vi "dataQ Terminal.vi"() -> ()   [LabVIEW 2024]
doc: "This example performs writes and reads on a serial port, as directed by the user. You can press the Write and Read buttons, and change the Read Count, while the example is running.\n\nThe parameters set for the serial port must match the parameters of the connected instrument or device. In this example, the Read Count parameter specifies the number of bytes that the serial port reads. If there were more bytes at the port than the specified number, those bytes would not be read. If there were less bytes at the port than the specified number, you would receive a timeout error.\n\nThis example expands upon the flow control options for XON and XOFF, allowing the user to choose those control characters. Also, the user can enable or disable a termination character. Some devices require a termination character in order to identify the end of command strings. Some devices send a termination character to signify the end of data to be read. This example shows how you can end the Read operation once a termination character is detected in the buffer and/or append a termination character at the end of the Write data."
uses:
  <vilib>/Instr/_visa.llb/VISA Configure Serial Port (Instr).vi
panel:
  out "Numeric":i32
  out "read buffer":string
  in  "Command List":string="stop\nencode 0\nslist 0 0\nslist 1 1\nsrate 6000\nps 2\ndec 1\ndeca 3\nnop\n"
  in  "2108 CDC Virtual COM":refnum<visa-resource-name>="COM3"
  # "Analog In\n\nencode 0\nslist 0 0\nslist 1 1\nsrate 6000\nps 2\ndec 1\ndeca 3\nnop"
  # "encode 0\nslist 0 0\nslist 1 1\nsrate 6000\nps 2\ndec 1\ndeca 3\nnop"
  # "encode 0 Enables the binary output mode (DEFAULT"
  # "info 0    Returns \"info 0 DATAQ\"\ninfo 1    Returns device model number (e.g.\"info 1 2008\")\ninfo 2    Returns firmware revision, 2 hex bytes (e.g. 6516 = 10110 for firmware revision 1.01)\ninfo 3    to info 4 Proprietary internal use for initial system verification\ninfo 5    <arg0>\n            Sets device description string arg0 (31 characters followed by null). Issued without <arg0> returns the \n            previously defined device description string. arg0 may be contained within quotation marks to included spaces \n            in device description. Model DI-2008 does not support info 5.\ninfo 6    Returns the instrument's serial number (left-most 8 digits only)\ninfo 7    to info 8 Proprietary internal use for initial system verification\ninfo 9    Returns the sample rate dividend value based upon current settings (see the srate command for details"
  # "0x60 = 96   FILL\n0x40 = 64  OFF\n0x20 = 32  DRAIN\n0x00 = 00  OFF"
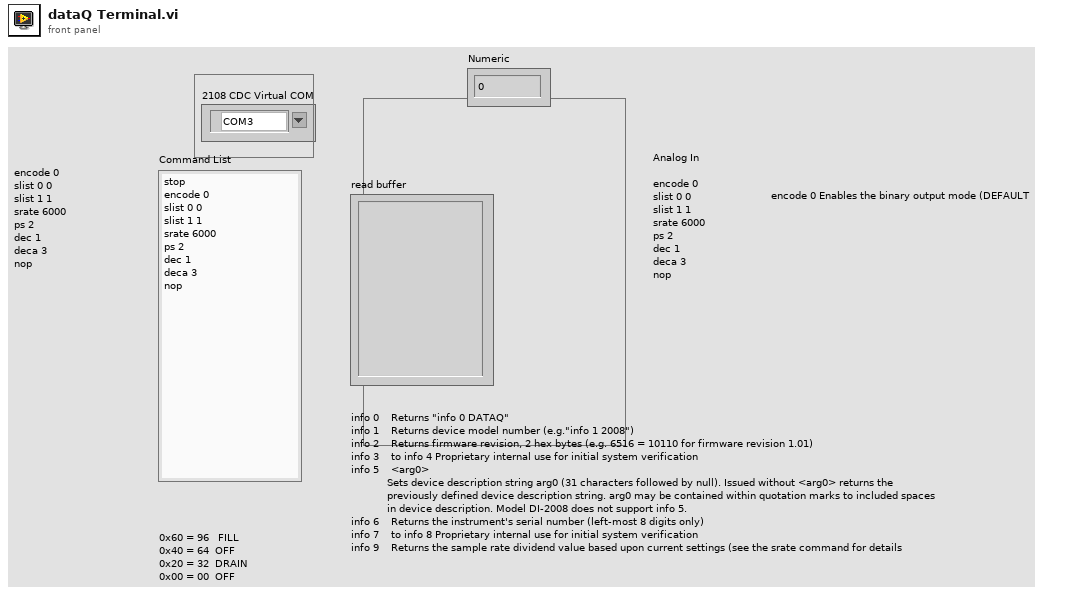
[diagram p1: front panel]
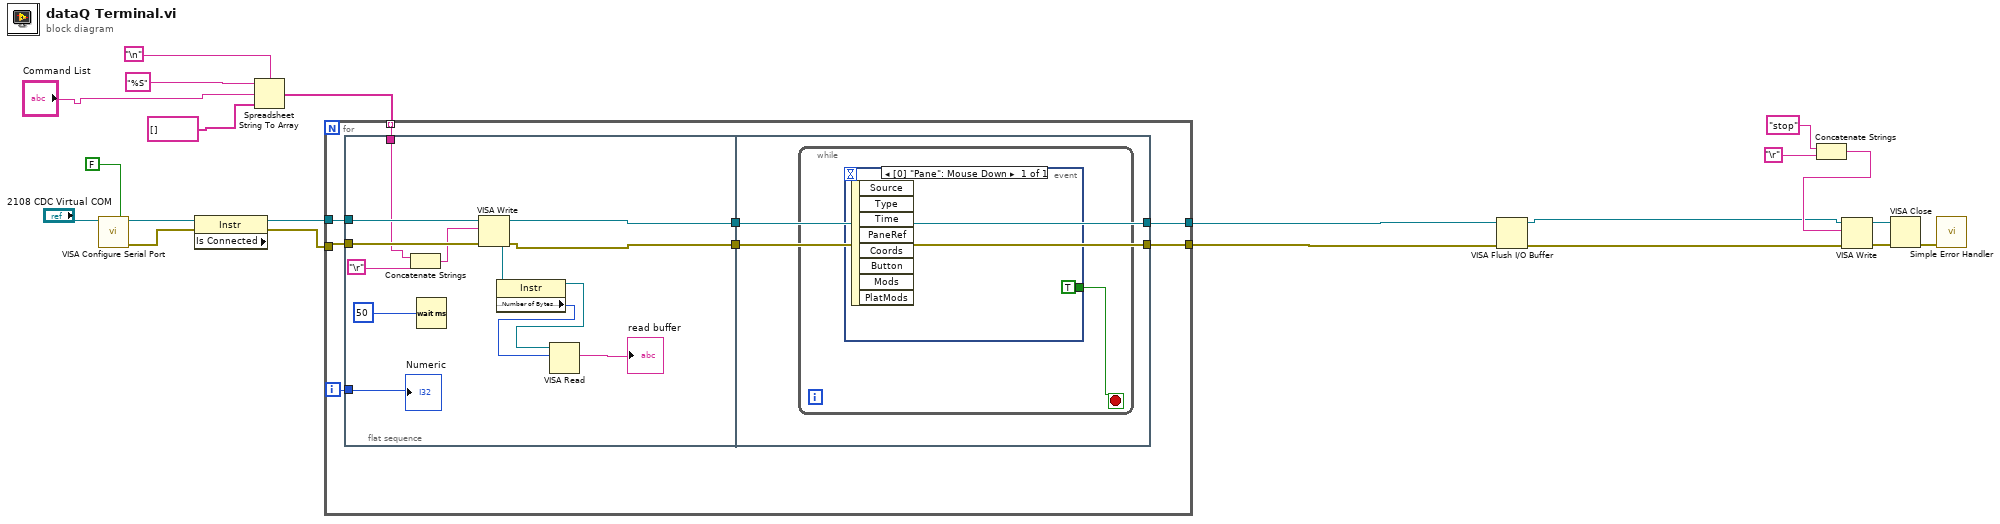
[diagram p0: block diagram]
diagram:
  n1 = call-poly "VISA Configure Serial Port"("VISA resource name"="2108 CDC Virtual COM", "Enable Termination\nChar (T)"=FALSE) -> ("VISA resource name out"=w19:refnum<visa-resource-name>, "error out"=w21:errorcluster)  [unwired: 8 in, 4 out]
  n2 = property class="Instr" props=["Is Connected"](reference=w19, error in=w21) -> (reference out=w5:refnum<visa-resource-name>, error out=w4:errorcluster)  [unwired: 1 out]
  n3 = Spreadsheet String To Array(delimiter (Tab)="\n", format string="%S", spreadsheet string="Command List", array type (2D Dbl)=string[] []) -> (array=w15:string[])
  n4 = for {
    tunnel: w15 -> [w27] mode=indexing
    tunnel: w5 -> [w29]
    tunnel: w4 -> [w28]
    tunnel: [w25] -> w7
    tunnel: [w26] -> w6
    i -> [w22]
    n5 = flat-sequence {
      tunnel: w29 -> [w41]
      tunnel: w28 -> [w40]
      tunnel: w27 -> [w38]
      tunnel: [w35] -> w24
      tunnel: [w34] -> w23
      tunnel: w22 -> [w30]
      tunnel: [w42] -> w25
      tunnel: [w43] -> w26
      tunnel: w24 -> [w43]
      tunnel: w23 -> [w42]
      frame #0 {
        n6 = Concatenate Strings(w38, "\r") -> (w36:string)
        n7 = Wait (ms)(milliseconds to wait=u32 50) -> ()  [unwired: 1 out]
        n8 = VISA Write(VISA resource name=w41, write buffer=w36, error in (no error)=w40) -> (VISA resource name out=w34:refnum<visa-resource-name>, error out=w35:errorcluster)  [unwired: 1 out]
        n9 = property class="Instr"(reference=w34) -> (reference out=w33:refnum<visa-resource-name>, "Serial Settings:Number of Bytes at Serial Port"=w32:u32)  [unwired: 1 in, 1 out]
        n10 = VISA Read(VISA resource name=w33, byte count=w32) -> (read buffer=→"read buffer":string)  [unwired: 1 in, 3 out]
        "Numeric" <- w30
      }
      frame #1 {
        n11 = while {
          stop <- w44 stop-if-true
          n12 = event shown="[0] \"Pane\": Mouse Down" {
            selector: _ -> [_]
            dyn-events: _ -> [_]
            timeout: _ -> [_]
            tunnel: [TRUE] -> w44
            event Mouse Down {
              n13 = event-data() -> ()  [unwired: 1 in, 8 out]
            }
          }
        }
      }
    }
  }
  n14 = VISA Flush I/O Buffer(VISA resource name=w7, error in (no error)=w6) -> (VISA resource name out=w2:refnum<visa-resource-name>, error out=w1:errorcluster)  [unwired: 1 in]
  n15 = Concatenate Strings("stop", "\r") -> (w9:string)
  n16 = VISA Write(VISA resource name=w2, write buffer=w9, error in (no error)=w1) -> (VISA resource name out=w13:refnum<visa-resource-name>, error out=w12:errorcluster)  [unwired: 1 out]
  n17 = VISA Close(VISA resource name=w13, error in (no error)=w12) -> (error out=w20:errorcluster)
  n18 = call <vilib>:"Simple Error Handler.vi"("error in (no error)"=w20) -> ()  [unwired: 1 in, 8 out]
